vi "Gateway(4800).vi"(5 "Принятый кадр":bool[](array[boolean]), 11 "Ошибка":bool) -> ()   [LabVIEW 2013]
panel:
  out "FER":dbl
  out "rate":dbl
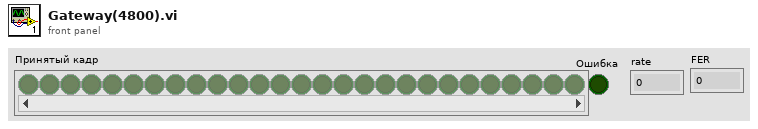
[diagram p1: front panel]
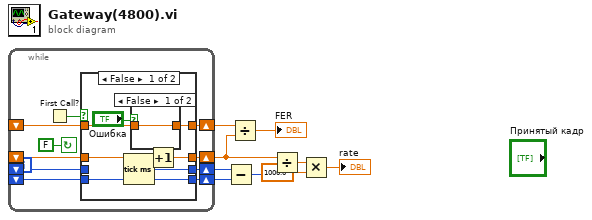
[diagram p0: block diagram]
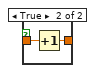
[diagram p2: hidden frame]
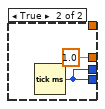
[diagram p3: hidden frame]
diagram:
  n1 = while {
    shift-right: [w17] -> w2
    shift-left: _ -> [w16]
    shift-right: [w15] -> w9
    shift-left: _ -> [w14]
    shift-right: [w13] -> w8
    shift-left: _ -> [w12]
    shift-right: [w11] -> w3
    shift-left: _ -> [w10]
    stop <- FALSE continue-if-true
    n2 = First Call?() -> (First Call?: T/F=w18:bool)
    n3 = case shown="False" w18 {
      tunnel: [w26 1.0] -> w17
      tunnel: w16 -> [w25 _]
      tunnel: [w24 w31] -> w15
      tunnel: w14 -> [w24 _]
      tunnel: [w23 w31] -> w13
      tunnel: w12 -> [_ _]
      tunnel: [w20 _] -> w11
      tunnel: w10 -> [w21 _]
      frame False {
        n4 = Tick Count (ms)() -> (millisecond timer value=w23:u32)
        n5 = case shown="False" "Ошибка" {
          tunnel: w21 -> [w27 w29]
          tunnel: [w27 w28] -> w20
          frame False {
          }
          frame True {
            n6 = Increment(x=w29) -> (x+1=w28:dbl)
          }
        }
        n7 = Increment(x=w25) -> (x+1=w26:dbl)
      }
      frame True {
        n8 = Tick Count (ms)() -> (millisecond timer value=w31:u32)
      }
    }
  }
  n9 = Subtract(x=w8, y=w9) -> (x-y=w7:u32)
  n10 = Divide(x=w3, y=w2) -> (x/y=→"FER":dbl)
  n11 = Divide(x=w2, y=w7) -> (x/y=w6:dbl)
  n12 = Multiply(x=w6, y=1000.0) -> (x*y=→"rate":dbl)
